vi "svx_Snd Write Waveform (DAQmx).vi"(0 "task ID":refnum<k21>, 1 "wave file path":path, 5 "waveform data":waveform(dbl)={"t0"=timestamp(0 s since 1904-01-01), "dt"=0.0, "Y"=[]}, 7 "bits per sample":i32=16, 11 "error in (no error)":errorcluster, 12 "sample rate [S/s]":enum16{"11025", "22050", "44100", "8000"}(ring)=enum."44100") -> (3 "dup wave file path":path, 4 "dup task ID":refnum<k21>, 6 "normalized data":waveform(dbl), 14 "SVT Wav info out":T1, 15 "error out":errorcluster)   [LabVIEW 2017]
uses:
  <resource>/objmgr/daqmx.rc
panel:
  in  "SVT Wav info":T1
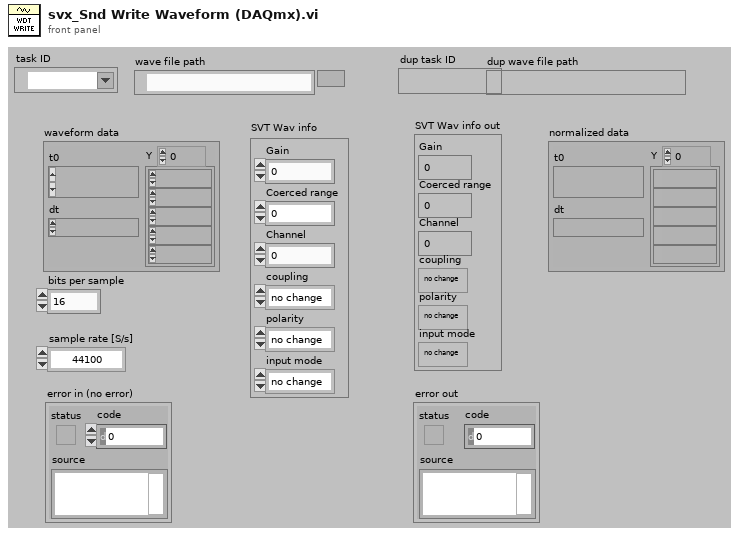
[diagram p1: front panel]
types:
  T1 = cluster{"Gain":u16, "Coerced range":u16, "Channel":u16, "coupling":enum16{"no change", "DC", "AC", "ground", "internal reference"}, "polarity":enum16{"no change", "bipolar", "unipolar"}, "input mode":enum16{"no change", "differential", "rse", "nrse"}}
  T2 = enum16{"no change", "DC", "AC", "ground", "internal reference"}
  T3 = enum16{"no change", "differential", "rse", "nrse"}
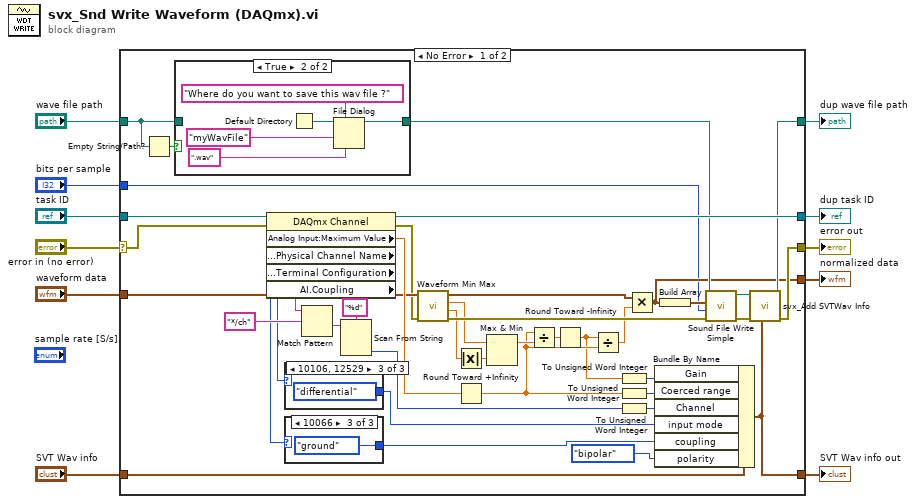
[diagram p0: block diagram]
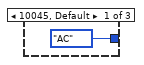
[diagram p2: hidden frame]
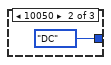
[diagram p3: hidden frame]
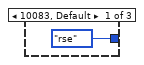
[diagram p4: hidden frame]
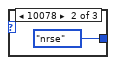
[diagram p5: hidden frame]
diagram:
  n1 = case shown="No Error" "error in (no error)" {
    selector: "error in (no error)" -> [w22 w68]
    tunnel: [w19 w66] -> w11
    tunnel: "SVT Wav info" -> [w52 w65]
    tunnel: [w51 w65] -> w9
    tunnel: "wave file path" -> [w49 w66]
    tunnel: "task ID" -> [w23 w67]
    tunnel: [w43 w67] -> w6
    tunnel: [w39 w68] -> w5
    tunnel: "waveform data" -> [w29 _]
    tunnel: [w13 _] -> w2
    tunnel: "bits per sample" -> [w12 _]
    frame No Error {
      n2 = Empty String/Path?(string/path=w49) -> (empty?=w50:bool)
      n3 = case shown="True" w50 {
        tunnel: w49 -> [w59 _]
        tunnel: [w59 w64] -> w20
        frame False {
        }
        frame True {
          n4 = Default Directory() -> (w62:path)
          n5 = File Dialog(6:".wav" ("pattern"), 7:"Where do you want to save this wav file ?" ("prompt"), 9:"myWavFile" ("default name"), 11:w62) -> (3:w64:path)  [unwired: 3 in, 3 out]
        }
      }
      n6 = property class="DAQmx Channel"(reference=w23, error in=w22) -> (reference out=w43:refnum<k21>, error out=w28:errorcluster, "Analog Input:Maximum Value"=w31:dbl, "General Properties:Physical Channel Name"=w48:tag, "Analog Input:General Properties:Input Configuration:Terminal Configuration"=w40:i32, "AI.Coupling"=w21:i32)
      n7 = case shown="10106, 12529" w40 {
        tunnel: [T3."rse" ("input mode") T3."nrse" ("input mode") T3."differential" ("input mode")] -> w18
        frame 10083, Default {
        }
        frame 10078 {
        }
        frame 10106, 12529 {
        }
      }
      n8 = case shown="10066" w21 {
        tunnel: [T2."AC" ("coupling") T2."DC" ("coupling") T2."ground" ("coupling")] -> w38
        frame 10045, Default {
        }
        frame 10050 {
        }
        frame 10066 {
        }
      }
      n9 = Match Pattern(string=w48, regular expression="*/ch") -> (after substring=w45:string)  [unwired: 1 in, 3 out]
      n10 = Scan From String(format string="%d" ("Format String"), input string=w45) -> (output 1=w44:i32)  [unwired: 3 in, 3 out]
      n11 = call <vilib>:"Waveform Min Max.vi"("error in (no error)"=w28, "waveform in"=w29) -> ("error out"=w27:errorcluster, "Y min"=w25:dbl, "Y max"=w26:dbl, "waveform out"=w15:waveform(dbl))  [unwired: 4 in, 2 out]
      n12 = Absolute Value(x=w25) -> (abs(x)=w34:dbl)
      n13 = Round Toward +Infinity(x=w31) -> (ceil(x): smallest int >= x=w17:dbl)
      n14 = Max & Min(x=w26, y=w34) -> (max(x,y)=w32:dbl)  [unwired: 1 out]
      n15 = Divide(x=w17, y=w32) -> (x/y=w33:dbl)
      n16 = Round Toward -Infinity(1:w33) -> (0:w14:dbl)
      n17 = Divide(x=w14, y=w17) -> (x/y=w16:dbl)
      n18 = To Unsigned Word Integer(number=w14) -> (unsigned 16bit integer=w24:u16)
      n19 = To Unsigned Word Integer(number=w17) -> (unsigned 16bit integer=w30:u16)
      n20 = To Unsigned Word Integer(number=w44) -> (unsigned 16bit integer=w42:u16)
      n21 = Multiply(x=w15, y=w16) -> (x*y=w13:waveform(dbl))
      n22 = Bundle By Name(cluster=w52, "Gain"=w24, "Coerced range"=w30, "Channel"=w42, "input mode"=w18, "coupling"=w38, "polarity"=enum16{"no change", "bipolar", "unipolar"}."bipolar") -> (w51:T1)
      n23 = Build Array(w13) -> (w35:waveform(dbl)[])
      n24 = call <vilib>:"Sound File Write Simple.vi"("error in (no error)"=w27, "bits per sample"=w12, "data"=w35, "path"=w20) -> ("error out"=w36:errorcluster, "path out"=w37:path)  [unwired: 6 in]
      n25 = call <vilib>:"svx_Add SVTWav Info.vi"("SVT WAV info"=w51, "error in (no error)"=w36, "wave file path in"=w37) -> ("error out"=w39:errorcluster, "wave file path"=w19:path)  [unwired: 7 in]
    }
    frame Error {
    }
  }
  "dup wave file path" <- w11
  "error out" <- w5
  "dup task ID" <- w6
  "SVT Wav info out" <- w9
  "normalized data" <- w2
